vi "Check for Value Change.vi"(7 "Force Write?":bool, 9 "New Data":dbl[](array[numeric]), 11 "Last Value Data":dbl[](array[numeric])) -> (1 "Value Change?":bool, 3 "Indices to Update":bool[](array[boolean]))   [LabVIEW 2020, in "Modbus Master Engine.lvlib"]
uses:
  Modbus Master Engine.lvlib
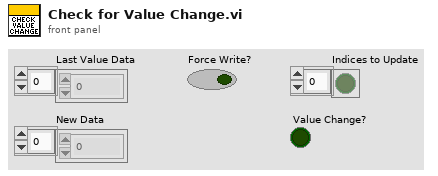
[diagram p1: front panel]
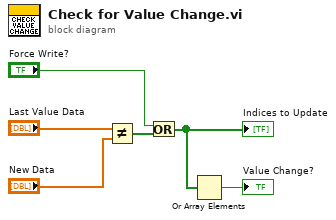
[diagram p0: block diagram]
diagram:
  n1 = Not Equal?(x="Last Value Data", y="New Data") -> (x != y?=w6:bool[])
  n2 = Or(x="Force Write?", y=w6) -> (x .or. y?=w2:bool[])
  "Indices to Update" <- w2
  n3 = Or Array Elements(Boolean array=w2) -> (logical OR=→"Value Change?":bool)
